vi "heartbeatReadCreate.vi"(8 "error in (no error)":errorcluster, 10 "interface object in":refnum<k20>, 11 "MotorControllerClass in":refnum<class "MotorControllerClass.lvclass">) -> (0 "error out":errorcluster, 1 "heartbeat object out":refnum<k20>, 2 "interface object out":refnum<k20>, 3 "MotorControllerClass out":refnum<class "MotorControllerClass.lvclass">)   [LabVIEW 2018, in "MotorControllerClass.lvclass"]
uses:
  BMS/MotorControllerClass.lvclass
  <vilib>/CANopenLib/CANOPEN.llb/CANopen Heartbeat Create.vi
  <vilib>/CANopenLib/CANOPEN.llb/CANopen Heartbeat Start.vi
panel:
  out "completion code":u32
  out "description":string
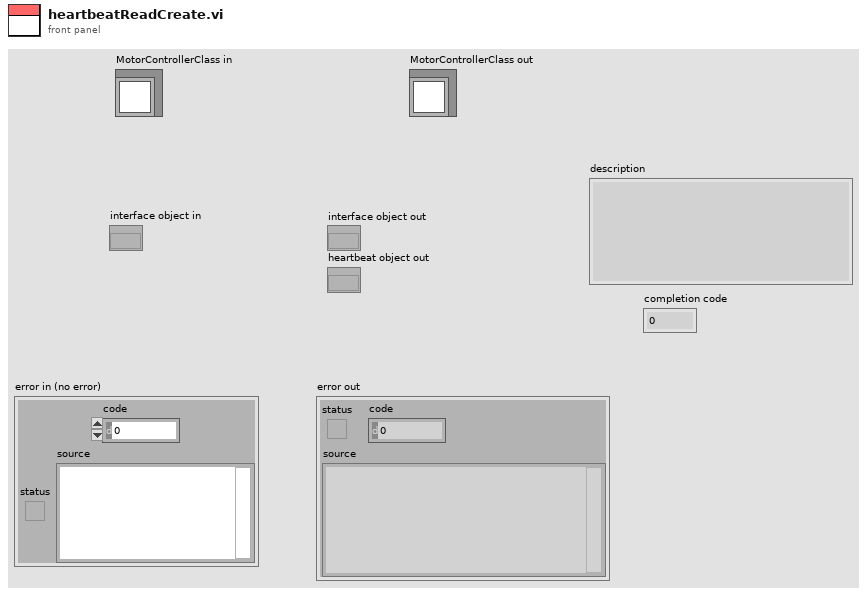
[diagram p1: front panel]
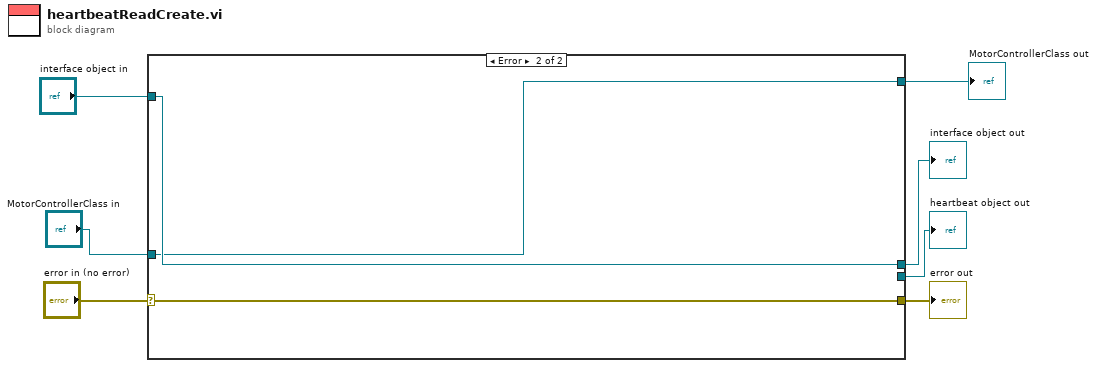
[diagram p0: block diagram]
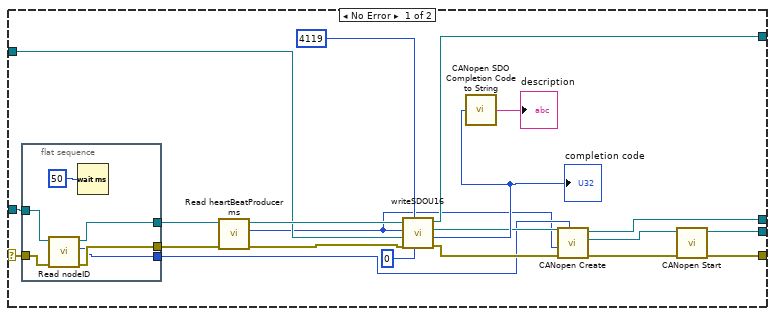
[diagram p2: hidden frame]
diagram:
  n1 = case shown="Error" "error in (no error)" {
    selector: "error in (no error)" -> [w27 w37]
    tunnel: [w24 w37] -> w6
    tunnel: "interface object in" -> [w18 w36]
    tunnel: [w25 _] -> w4
    tunnel: [w23 w36] -> w3
    tunnel: "MotorControllerClass in" -> [w21 w35]
    tunnel: [w12 w35] -> w1
    frame No Error {
      n2 = flat-sequence {
        tunnel: w27 -> [w31]
        tunnel: w21 -> [w33]
        tunnel: [w32] -> w20
        tunnel: [w30] -> w15
        tunnel: [w29] -> w9
        frame #0 {
          n3 = call-dynamic "Read nodeID.vi"("error in (no error)"=w31, "MotorControllerClass in"=w33) -> ("error out"=w30:errorcluster, "nodeID"=w29:u8, "MotorControllerClass out"=w32:refnum<class "MotorControllerClass.lvclass">)  [unwired: 7 in]
          n4 = Wait (ms)(milliseconds to wait=u32 50) -> ()  [unwired: 1 out]
        }
      }
      n5 = call-dynamic "Read heartBeatProducer ms.vi"("error in (no error)"=w15, "MotorControllerClass in"=w20) -> ("error out"=w14:errorcluster, "heartBeatProducer ms"=w8:u16, "MotorControllerClass out"=w19:refnum<class "MotorControllerClass.lvclass">)  [unwired: 7 in]
      n6 = call "writeSDOU16.vi"("object sub-index (0)"=u8 0, "object index"=u16 4119, "error in (no error)"=w14, "interface object in"=w18, "inputNumber"=w8, "MotorControllerClass in"=w19) -> ("error out"=w13:errorcluster, "completion code"=w11:u32, "interface object out"=w10:refnum<k20>, "MotorControllerClass out"=w12:refnum<class "MotorControllerClass.lvclass">)  [unwired: 2 in]
      "completion code" <- w11
      n7 = call <vilib>:"CANopen SDO Completion Code to String.vi"("SDO completion code"=w11) -> ("description"=→"description":string)
      n8 = call-poly <vilib>:"CANopen Create.vi"("node-ID"=w9, "error in (no error)"=w13, "consumer time [ms]"=w8, "interface object in"=w10) -> ("error out"=w28:errorcluster, "heartbeat object out"=w26:refnum<k20>, "interface object out"=w23:refnum<k20>)  [unwired: 5 in]
      n9 = call-poly <vilib>:"CANopen Start.vi"("error in (no error)"=w28, "heartbeat object in"=w26) -> ("error out"=w24:errorcluster, "heartbeat object out"=w25:refnum<k20>)  [unwired: 8 in]
    }
    frame Error {
    }
  }
  "error out" <- w6
  "interface object out" <- w3
  "heartbeat object out" <- w4
  "MotorControllerClass out" <- w1
